vi "testRSASign&VerifyInvalidSignature.vi"(8 "error in (no error)":errorcluster, 11 "TestCase in":refnum<class "TestRSA.lvclass">) -> (0 "error out":errorcluster, 3 "TestCase out":refnum<class "TestRSA.lvclass">)   [LabVIEW 2021, in "TestRSA.lvclass"]
uses:
  TestRSA.lvclass
  Source Code/Utility/HashingAlgorithm.ctl
  Source Code/Asymmetric Encryption/RSASignaturePadding.ctl
  <vilib>/addons/_JKI Toolkits/VI Tester/TestCase.llb/TestCase.lvclass
  Source Code/Asymmetric Encryption/dotNET Crypto Asymmetric Encryption.lvlib
  Source Code/Key Management/dotNET Crypto Key Management.lvlib
  Source Code/Utility/dotNET Crypto Utility.lvlib
  C:/Program Files (x86)/National Instruments/LabVIEW 2021/vi.lib/addons/_JKI Toolkits/VI Tester/TestCase.llb/TestCase.lvclass
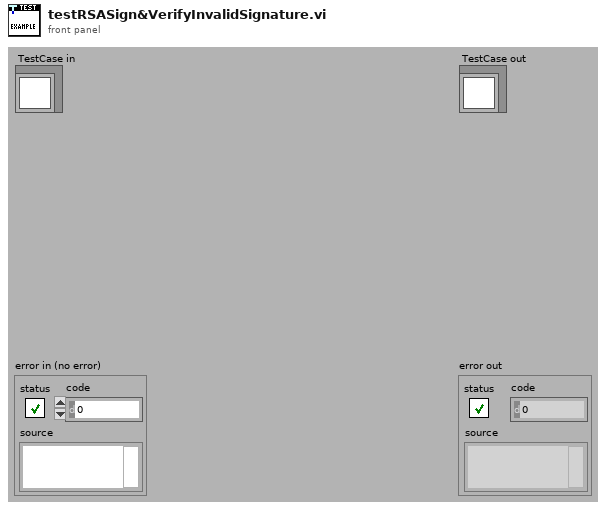
[diagram p1: front panel]
types:
  T1 = typedef "dotNET Crypto Asymmetric Encryption.lvlib/RSASignaturePadding.ctl" = enum16{"Pkcs1", "Pss"}
  T2 = typedef "dotNET Crypto Utility.lvlib/HashingAlgorithm.ctl" = enum16{"MD5", "SHA1", "SHA256", "SHA384", "SHA512"}
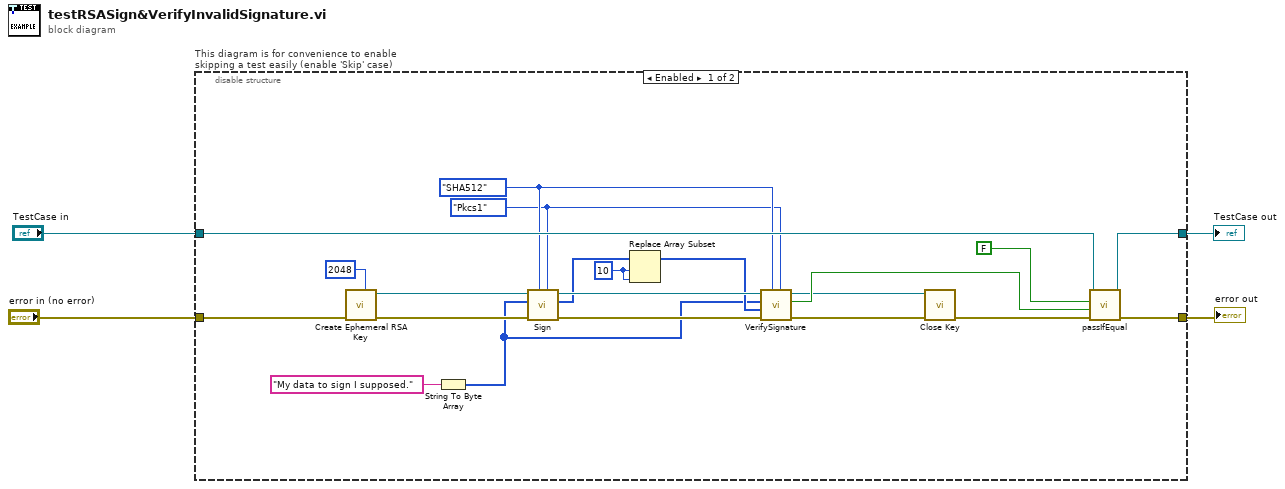
[diagram p0: block diagram]
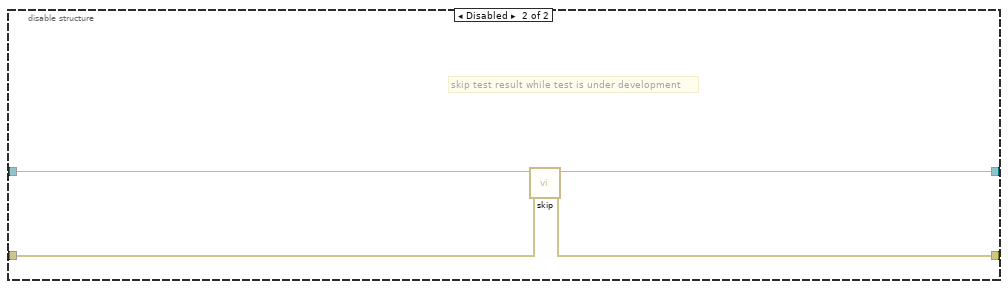
[diagram p2: hidden frame]
diagram:
  n1 = disable-structure "This diagram is for convenience to enable skipping a test easily (enable 'Skip' case)" shown="Enabled" {
    disable-tunnel: "TestCase in" -> [w25 w29]
    disable-tunnel: [w24 w27] -> w1
    disable-tunnel: [w23 w28] -> w3
    disable-tunnel: "error in (no error)" -> [w22 w26]
    frame Enabled {
      w14 = 10 ("index")
      w18 = RSASignaturePadding."Pkcs1" ("RSASignPadding")
      w19 = HashingAlgorithm."SHA512" ("HashingAlgorithm")
      n2 = call "Create Ephemeral RSA Key.vi"("Key Length (2048)"=2048 ("keySize (2048 bit)"), "error in (no error)"=w22) -> ("error out"=w21:errorcluster, "CngKey out"=w9:refnum<k24>)  [unwired: 8 in]
      n3 = String To Byte Array(string="My data to sign I supposed.") -> (unsigned byte array=w10:u8[])
      n4 = call "Sign.vi"("RSASignPadding"=w18, "HashingAlgorithm"=w19, "error in (no error)"=w21, "Data in"=w10, "CngKey in"=w9) -> ("error out"=w20:errorcluster, "Signature out"=w12:u8[], "CngKey out"=w13:refnum<k24>)  [unwired: 4 in]
      n5 = Replace Array Subset(array=w12, new element=w14, index=w14) -> (w11:u8[])
      n6 = call "VerifySignature.vi"("RSASignPadding"=w18, "HashingAlgorithm"=w19, "error in (no error)"=w20, "Signature in"=w11, "Data in"=w10, "CngKey in"=w13) -> ("error out"=w17:errorcluster, "Verified?"=w7:bool, "CngKey out"=w5:refnum<k24>)  [unwired: 3 in]
      n7 = call "Close Key.vi"("error in (no error)"=w17, "CngKey in"=w5) -> ("error out"=w6:errorcluster)  [unwired: 9 in]
      n8 = call-dynamic "passIfEqual.vi"("error in (no error)"=w6, "y"=w7, "x"=FALSE, "TestCase in"=w25) -> ("error out"=w23:errorcluster, "TestCase out"=w24:refnum<class "TestRSA.lvclass">)  [unwired: 6 in]
    }
    frame Disabled {
      # "skip test result while test is under development"
      n9 = call <vilib>:"skip.vi"("error in (no error)"=w26, "TestCase in"=w29) -> ("error out"=w28:errorcluster, "TestCase out"=w27:refnum<class "TestRSA.lvclass">)  [unwired: 8 in]
    }
  }
  "error out" <- w3
  "TestCase out" <- w1
